vi "Get Gate Status.vi"(8 "error in (no error)":errorcluster, 11 "gate":T1) -> (0 "error out":errorcluster, 1 "# waiting for open gate":i32, 2 "gate name":string, 3 "gate out":T1)   [LabVIEW 2015, in "Gates.lvlib"]
doc: "Returns current status information of a gate."
uses:
  Gates.lvlib
  Gate.ctl
  Gate Pass.ctl
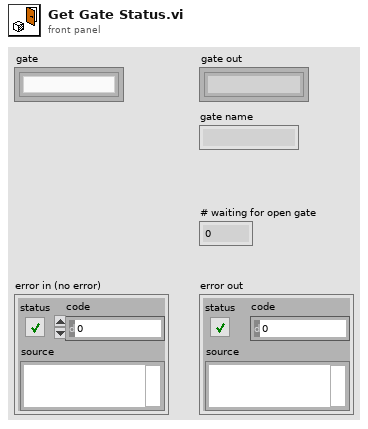
[diagram p1: front panel]
types:
  T1 = typedef "Gates.lvlib/Gate.ctl" = refnum<k1>
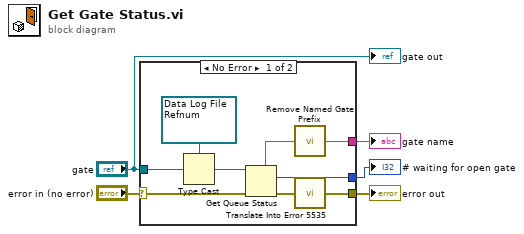
[diagram p0: block diagram]
diagram:
  n1 = case shown="No Error" "error in (no error)" {
    selector: "error in (no error)" -> [w10 w15]
    tunnel: [w14 w15] -> w5
    tunnel: [w6 _] -> w4
    tunnel: "gate" -> [w11 _]
    tunnel: [w9 _] -> w1
    frame No Error {
      w12 = refnum<queue> refnum items=["Gate Pass"] ("queue out")
      n2 = Type Cast(type=w12, x=w11) -> (*(type *) &x=w13:refnum<queue>)
      n3 = Get Queue Status(queue=w13, error in (no error)=w10) -> (queue name=w8:string, # pending remove=w6:i32, error out=w7:errorcluster)  [unwired: 1 in, 5 out]
      n4 = call "Remove Named Gate Prefix.vi"("name in"=w8) -> ("name out"=w9:string)
      n5 = call "Translate Into Error 5535.vi"("error in (no error)"=w7) -> ("error out"=w14:errorcluster)  [unwired: 1 in]
    }
    frame Error {
    }
  }
  "error out" <- w5
  "# waiting for open gate" <- w4
  "gate name" <- w1
  "gate out" <- "gate"
